vi "_TCP Msg Read.vi"(8 "error in":errorcluster, 9 "Ignore Timeout Error (T)":bool=TRUE, 10 "timeout ms (10000)":i32=10000, 11 "connection ID":refnum<k5>) -> (0 "error out":errorcluster, 1 "Message Type":string, 2 "Data Stream":string, 3 "connection ID out":refnum<k5>, 4 "Data Size":i32, 5 "Timed Out?":bool, 6 "Checksum":u16)   [LabVIEW 2015]
doc: "Reads an incoming package of data from a remote host via TCP/IP. This VI parses the package and extracts the data name and type as described in the meta data.\n\nFor the package to be parsed correctly, the meta data must be consistent in both the sender and the receiver. The data is packaged based on the existing meta data on the sender. Inconsistent meta data will result in inconsistent data parsing.\nUse the \"Read Meta\" and \"Write Meta\" VIs to ensure that both client and server have the same meta data.\n\nThe data is returned as a string. It is the responsibility of the user to cast it to the appropriate type before usage."
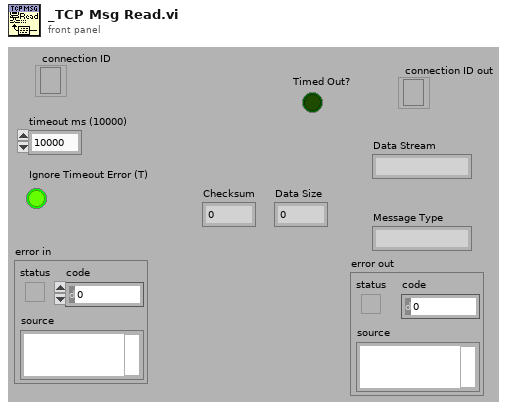
[diagram p1: front panel]
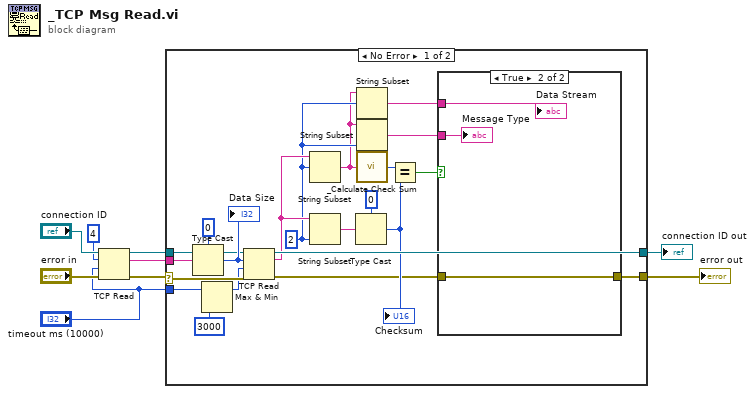
[diagram p0: block diagram]
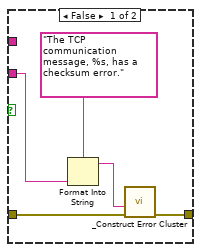
[diagram p2: hidden frame]
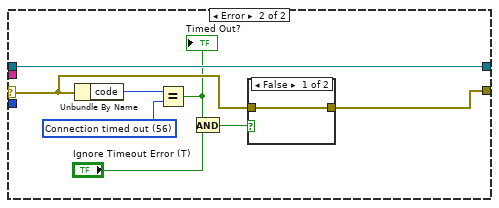
[diagram p3: hidden frame]
diagram:
  n1 = TCP Read(connection ID="connection ID", bytes to read=4, error in (no error)="error in", 9:"timeout ms (10000)") -> (connection ID out=w5:refnum<k5>, data out=w6:string, error out=w3:errorcluster)  [unwired: 1 out]
  n2 = case shown="No Error" w3 {
    selector: w3 -> [w25 w41]
    tunnel: w6 -> [w30 _]
    tunnel: w5 -> [w27 w46]
    tunnel: "timeout ms (10000)" -> [w11 _]
    tunnel: [w24 w46] -> w2
    tunnel: [w15 w42] -> w1
    frame No Error {
      w19 = 2 ("length (rest)")
      n3 = Type Cast(type=0 ("bytes to read"), x=w30) -> (*(type *) &x=w28:i32)
      "Data Size" <- w28
      n4 = Max & Min(x=w11, y=3000) -> (max(x,y)=w10:i32)  [unwired: 1 out]
      n5 = TCP Read(connection ID=w27, bytes to read=w28, error in (no error)=w25, 9:w10) -> (connection ID out=w24:refnum<k5>, data out=w22:string, error out=w16:errorcluster)  [unwired: 1 out]
      n6 = String Subset(string=w22, offset (0)=w19) -> (substring=w18:string)  [unwired: 1 out]
      n7 = String Subset(string=w22, length (rest)=w19) -> (substring=w23:string)  [unwired: 1 out]
      n8 = Type Cast(type=u16 0 ("bytes to read"), x=w23) -> (*(type *) &x=w20:u16)
      "Checksum" <- w20
      n9 = String Subset(string=w18, offset (0)=w19) -> (substring=w13:string)  [unwired: 1 out]
      n10 = String Subset(string=w18, length (rest)=w19) -> (substring=w14:string)  [unwired: 1 out]
      n11 = call "_Calculate Check Sum.vi"("Stream"=w18) -> ("Checksum"=w21:u16)
      n12 = Equal?(x=w21, y=w20) -> (x = y?=w17:bool)
      n13 = case shown="True" w17 {
        tunnel: w16 -> [w33 w38]
        tunnel: [w32 w38] -> w15
        tunnel: w14 -> [w35 w37]
        tunnel: w13 -> [_ w36]
        frame False {
          n14 = Format Into String(format string="The TCP communication message, %s, has a checksum error.", w35) -> (resulting string=w31:string)  [unwired: 2 in, 1 out]
          n15 = call "_Construct Error Cluster.vi"("error in"=w33, "reason"=w31) -> ("error out"=w32:errorcluster)  [unwired: 2 in, 3 out]
        }
        frame True {
          "Message Type" <- w37
          "Data Stream" <- w36
        }
      }
    }
    frame Error {
      w44 = 56 items=["No Error", "Argument Error", "Memory Full", "Out of Zone", "End of File", "File Already Open", "Generic File IO Error", "File Not Found", "File Permission Error", "Disk Full", "Duplicate Path", "Too Many Files Open", "Not Enabled", "Resource File Not Found", "Cannot Add Resource", "Resource Not Found", "Image Not Found", "Image Memory Error", "Pen Does Not Exist", "Config Bad Type", "Config Token Not Found", "Config Parse Error", "Config Memory Error", "Bad External Code Format", "Bad External Code Offset", "External Code Not Present", "Null Window", "Destroy Window Mixup", "Null Menu", "Print Aborted", "Bad Print Record", "Print Driver Error", "Windows Error During Print", "Memory Error During Print", "Print Dialog Error", "Generic Print Error", "Invalid Device Refnum", "Device Not Found", "Device Parameter Error", "Device Unit Error", "Can't Open Device", "Device Call Aborted", "Generic Error", "Cancelled By User", "Object ID Too Low", "Object ID Too High", "Object Not In Heap", "Unknown Heap", "Bad DefProc ID", "DefProc Not In Table", "Message Out Of Range", "Null Method", "Unknown Message", "Manager Call Not Supported", "Bad address", "Connection In progress", "Connection timed out", "Connection is already in progress", "Network attribute not supported", "Network error", "Address in use", "System out of memory", "Connection aborted", "Connection refused", "Connection is not connected", "Connection is already connected", "Connection closed", "Initialize error (interapplication manager)", "Bad occurrence", "Wait on unbound occurrence handler", "Occurrence queue overflow", "Bad path", "Semaphore not signaled", "Unrecognized type (interapplication manager)"] ("1st Error to Convert")
      n16 = Unbundle By Name(w41) -> ("code"=w45:i32)
      n17 = Equal?(x=w45, y=w44) -> (x = y?=w40:bool)
      "Timed Out?" <- w40
      n18 = And(x=w40, y="Ignore Timeout Error (T)") -> (x .and. y?=w43:bool)
      n19 = case shown="False" w43 {
        tunnel: [w47 _] -> w42
        tunnel: w41 -> [w47 _]
        frame False {
        }
        frame True {
        }
      }
    }
  }
  "error out" <- w1
  "connection ID out" <- w2
